vi "SYST_MACR_COPY_CHAN_TO.vi"(0 "VISA IN":refnum<visa-resource-name>, 1 "Target":i32, 5 "error in":errorcluster, 7 "Source":i32) -> (14 "VISA Out":refnum<visa-resource-name>, 19 "error out":errorcluster)   [LabVIEW 2018, in "PNA-X.lvlib"]
doc: "SYSTem:MACRo:COPY:CHANnel<cnum>[:TO] <num> \n1875\n\n(Write-only) Sets up channel <num> as a copy of channel <cnum>. Learn more about copy channels. \nParameters \n<cnum> Any existing channel number. If unspecified, value is set to 1. \n<num> Number of the channel which is to become a copy of channel <cnum>. \nExamples SYST:MACR:COPY:CHAN1 2 \nsystem:macro:copy:channel2:to 3 \nQuery Syntax Not Applicable \nDefault Not Applicable"
uses:
  PNA-X.lvlib
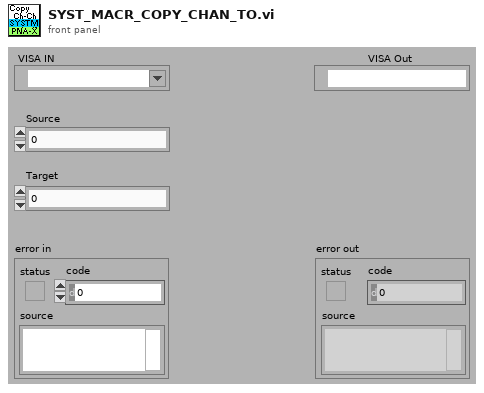
[diagram p1: front panel]
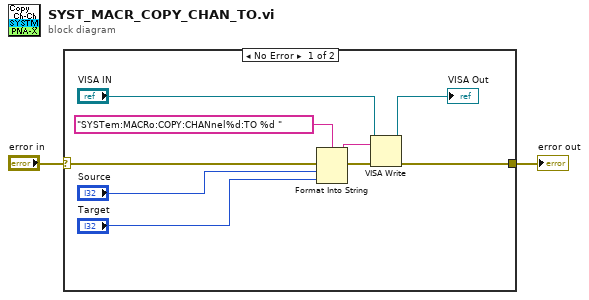
[diagram p0: block diagram]
diagram:
  n1 = case shown="No Error" "error in" {
    selector: "error in" -> [w11 w12]
    tunnel: [w6 w12] -> w1
    frame No Error {
      n2 = Format Into String(format string="SYSTem:MACRo:COPY:CHANnel%d:TO %d " ("Cmdline"), error in=w11, "Source", "Target") -> (resulting string=w9:string, error out=w10:errorcluster)  [unwired: 1 in]
      n3 = VISA Write(VISA resource name="VISA IN", write buffer=w9, error in (no error)=w10) -> (VISA resource name out=→"VISA Out":refnum<visa-resource-name>, error out=w6:errorcluster)  [unwired: 1 out]
    }
    frame Error {
    }
  }
  "error out" <- w1
